vi "Result All Steps Output Meter Readings.vi"() -> ()   [LabVIEW 2025]
uses:
  <instrlib>/Chroma 19052/Chroma 19052.lvlib
panel:
  out "VISA resource name out":refnum<visa-resource-name>
  in  "VISA resource name":refnum<visa-resource-name>
  out "error out":errorcluster
  in  "error in (no error)":errorcluster
  out "Results":string
  # "All Steps Output Meter Readings Result"
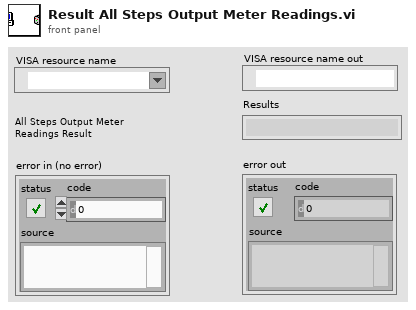
[diagram p1: front panel]
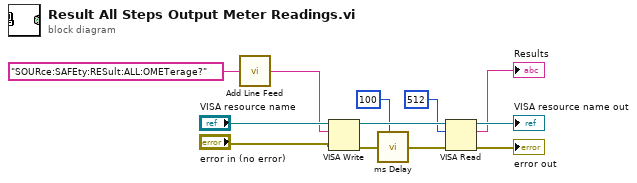
[diagram p0: block diagram]
diagram:
  n1 = call <instrlib>:"Add Line Feed.vi"("Command string"="SOURce:SAFEty:RESult:ALL:OMETerage?") -> ("Concatenated string"=w6:string)  [unwired: 4 in]
  n2 = VISA Write(VISA resource name="VISA resource name", write buffer=w6, error in (no error)="error in (no error)") -> (VISA resource name out=w12:refnum<visa-resource-name>, error out=w4:errorcluster)  [unwired: 1 out]
  n3 = call <instrlib>:"ms Delay.vi"("miliseconds to wait"=u32 100, "error in (no error)"=w4) -> ("error out"=w3:errorcluster)  [unwired: 6 in, 1 out]
  n4 = VISA Read(VISA resource name=w12, byte count=u32 512, error in (no error)=w3) -> (VISA resource name out=→"VISA resource name out":refnum<visa-resource-name>, read buffer=→"Results":string, error out=→"error out":errorcluster)  [unwired: 1 out]
